vi "Auto Iterate.vi"(11 "Hello World Event in":refnum<class "Hello World Event.lvclass">) -> (3 "Hello World Event out":refnum<class "Hello World Event.lvclass">)   [LabVIEW 2021, in "Hello World Event.lvlib" / "Hello World Event.lvclass"]
uses:
  Hello World Event.lvclass
  Hello World Event.lvclass/Hello World Event.ctl
  Auto Iterate Msg Strategy/Auto Iterate Msg Strategy.lvlib
  <vilib>/Nathan Davis/jettl/jettl/Msg Strategy/Msg Strategy.lvclass
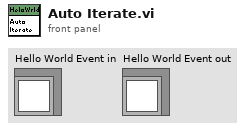
[diagram p1: front panel]
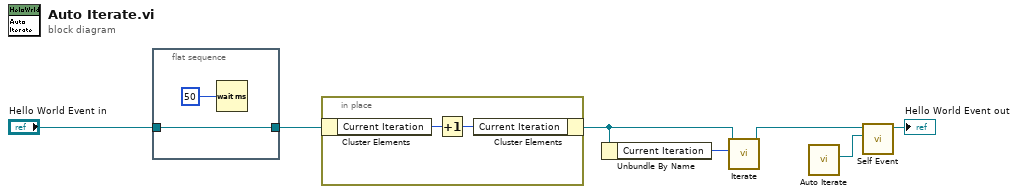
[diagram p0: block diagram]
diagram:
  n1 = flat-sequence {
    tunnel: [w8] -> w2
    tunnel: "Hello World Event in" -> [w8]
    frame #0 {
      n2 = Wait (ms)(milliseconds to wait=u32 50) -> ()  [unwired: 1 out]
    }
  }
  n3 = in-place {
    n4 = in-place-cluster #1(w2) -> ("Current Iteration"=w11:i32)
    n5 = Increment(x=w11) -> (x+1=w10:i32)
    n6 = in-place-cluster #1("Current Iteration"=w10) -> (w6:refnum<class "Hello World Event.lvclass">)
  }
  n7 = Unbundle By Name(w6) -> ("Current Iteration"=w5:i32)
  n8 = call-dynamic "Iterate.vi"("Iterate"=w5, "Hello World Event in"=w6) -> ("Hello World Event out"=w7:refnum<class "Hello World Event.lvclass">)  [unwired: 9 in]
  n9 = call "Auto Iterate.vi"() -> ("Msg Strategy"=w3:refnum<class "Msg Strategy.lvclass">)  [unwired: 11 in]
  n10 = call-dynamic "Self Event.vi"("Msg Strategy"=w3, "Hello World Event in"=w7) -> ("Hello World Event out"=→"Hello World Event out":refnum<class "Hello World Event.lvclass">)  [unwired: 9 in]
